vi "Sellafield_Stack_Changeover.vi"(3 "Mode":T5, 5 "Traverse line In":T2 {"Row Duration (mins)" format="%#.1f"; "Row No" min=0; "Trace Gas Concentration (%)" min=0.0 format="%#.2f"; "Emission Rate (l/min)" format="%#.2f"; "Tunnel Speed" format="%#.2f"; "Start X" format="%#.2f"; "Start Y" format="%#.2f"; "Start Z" format="%#.2f"; "End X" format="%#.2f"; "End Y" format="%#.2f"; "End Z" format="%#.2f"; "Averaging time (min)" min=0.0 format="%#.2f"}) -> (0 "Error Message":string, 1 "Status":T1, 2 "Traverse line Out":T2 {"Row Duration (mins)" format="%#.1f"; "Row No" min=0; "Trace Gas Concentration (%)" min=0.0 format="%#.2f"; "Emission Rate (l/min)" format="%#.2f"; "Tunnel Speed" format="%#.2f"; "Start X" format="%#.2f"; "Start Y" format="%#.2f"; "Start Z" format="%#.2f"; "End X" format="%#.2f"; "End Y" format="%#.2f"; "End Z" format="%#.2f"; "Averaging time (min)" min=0.0 format="%#.2f"})   [LabVIEW 2010]
uses:
  Gen Trav/Traverse_cluster.ctl
  Gen Trav/Spacing.ctl
  Controls/Multi_run_mode.ctl
  Controls/User_Specific_mode.ctl
  Gen Trav/Multi_Run_Status.ctl
  ADAM Client/Sub VIs/ADAM Controls/Update_scan_value.ctl
panel:
  # "X           Y            Z"
  # "Start"
  # "End"
  # "X           Y            Z"
  # "Start"
  # "End"
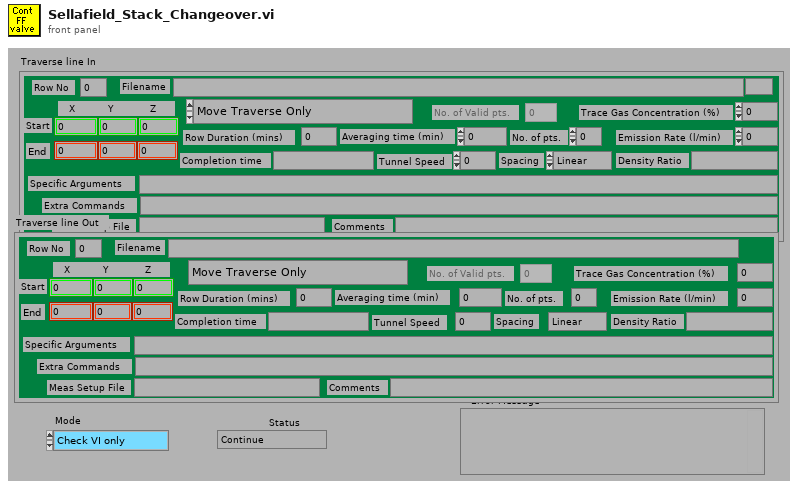
[diagram p1: front panel]
types:
  T1 = typedef "Multi_Run_Status.ctl" = enum16{"Continue", "Jump to Next Point", "Jump to Next Row", "Jump To Fall Back", "Terminate Run"}
  T2 = typedef "Traverse_cluster.ctl" = cluster{"Start X":dbl, "Start Y":dbl, "Start Z":dbl, "End X":dbl, "End Y":dbl, "End Z":dbl, "No. of pts.":i32, "Spacing":T3, "Filename":path, "Tunnel Speed":dbl, "Averaging time (min)":dbl, "Extra Commands":string, "Specific Arguments":string, "Emission Rate (l/min)":dbl, "Trace Gas Concentration (%)":dbl, "Density Ratio":string, "Comments":string, "Row No":i32, "Row Type Selector":T4, "Completion time":string, "Row Duration (mins)":dbl, "No. of Valid pts.":i32, "Meas Setup File":string}
  T3 = typedef "Spacing.ctl" = enum16{"Linear", "Log", "Gauss", "Specified", "N/A"}
  T4 = typedef "Multi_run_mode.ctl" = enum16{"Move Traverse Only", "Set Tunnel Speed Only", "Set Source Only", "Set Measurement Conditions", "Single Measurement", "Vertical Profile", "Lateral Profile", "Longitudinal Profile", "Explore Volume", "Multi-Axis Profile", "Auto Calibrate", "Meas Fast FID Bkgnd", "Check Beam Power", "Scanning Valve Measurement", "Run VI Named:", "Set ADAM Ch", "Wait (minutes)", "Send Message", "Synchronize With:", "Fall Back to this Row", "Turn Off Row Repeating", "Blank Row"}
  T5 = typedef "User_Specific_mode.ctl" = enum16{"Check VI only", "Run VI"}
  T6 = typedef "Update_scan_value.ctl" = cluster{"Channel Name":string, "New Value":dbl}
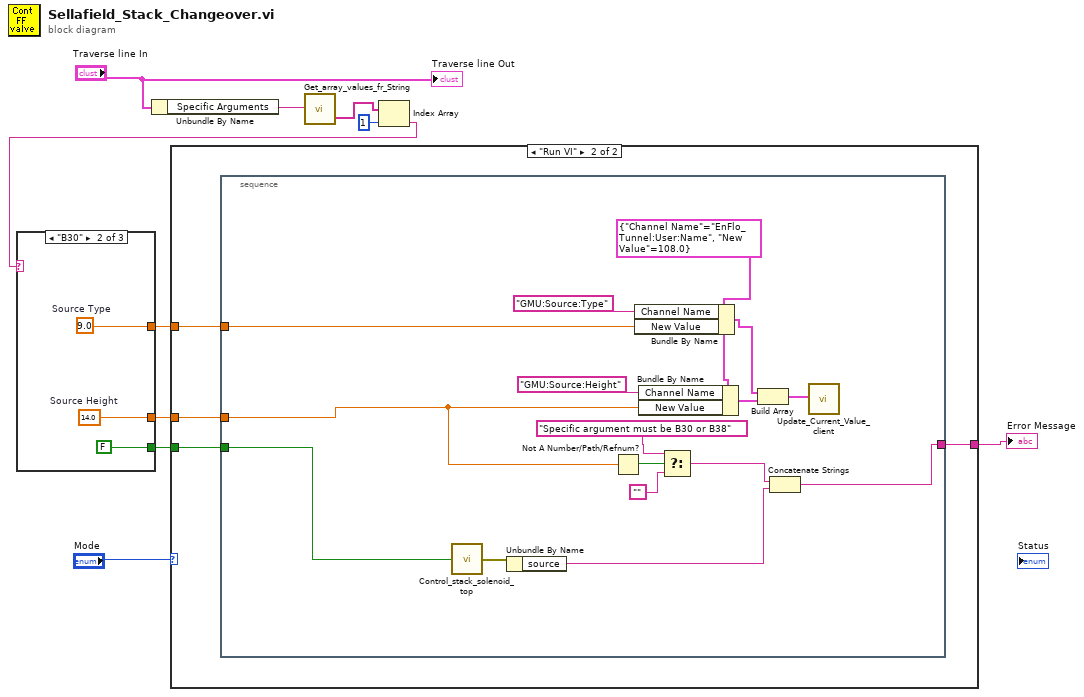
[diagram p0: block diagram]
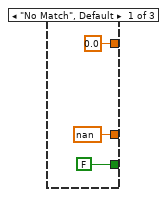
[diagram p2: hidden frame]
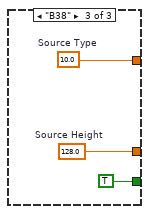
[diagram p3: hidden frame]
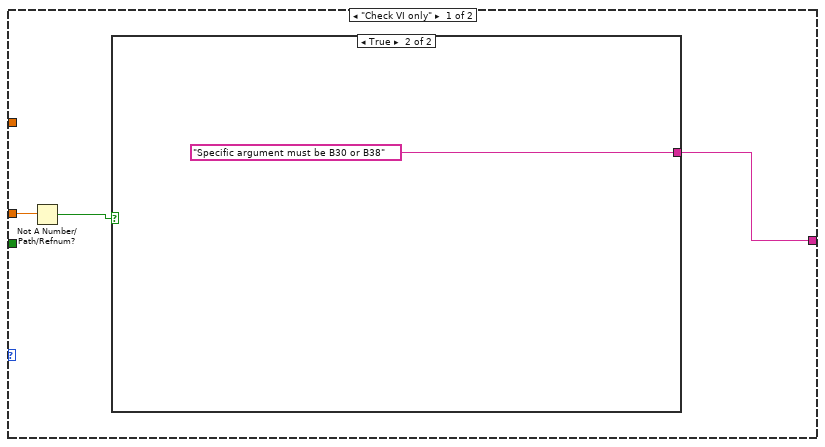
[diagram p4: hidden frame]
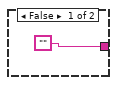
[diagram p5: hidden frame]
diagram:
  n1 = Unbundle By Name("Traverse line In") -> ("Specific Arguments"=w8:string)
  n2 = call "Get_array_values_fr_String.vi"("String Value"=w8) -> ("String array"=w7:string[])  [unwired: 1 out]
  n3 = Index Array(array=w7, index=1 ("Index")) -> (element=w5:string)
  n4 = case shown="\"B30\"" w5 {
    tunnel: [nan ("Source Height") w16 w19] -> w4
    tunnel: [0.0 ("Source Type") w15 w18] -> w3
    tunnel: [FALSE FALSE TRUE] -> w1
    frame "No Match", Default {
    }
    frame "B30" {
      w15 = 9.0  # Source Type
      w16 = 14.0  # Source Height
    }
    frame "B38" {
      w18 = 10.0  # Source Type
      w19 = 128.0  # Source Height
    }
  }
  n5 = case shown="\"Run VI\"" "Mode" {
    tunnel: w4 -> [w22 w28]
    tunnel: w3 -> [_ w27]
    tunnel: [w20 w25] -> w2
    tunnel: w1 -> [_ w26]
    frame "Check VI only" {
      n6 = Not A Number/Path/Refnum?(number/path/refnum=w22) -> (NaN/Path/Refnum?=w21:bool)
      n7 = case shown="True" w21 {
        tunnel: ["" "Specific argument must be B30 or B38"] -> w20
        frame False {
        }
        frame True {
        }
      }
    }
    frame "Run VI" {
      n8 = stacked-sequence {
        tunnel: w28 -> [w35]
        tunnel: w27 -> [w38]
        tunnel: w26 -> [w33]
        tunnel: [w29] -> w25
        frame #0 {
          w39 = T6 {"Channel Name"="EnFlo_Tunnel:User:Name", "New Value"=108.0} ("Update Scan Value Cluster")
          n9 = call "Control_stack_solenoid_top.vi"("Valve On?"=w33) -> ("s? t:f"=w32:errorcluster)  [unwired: 1 out]
          n10 = Unbundle By Name(w32) -> ("source"=w30:string)
          n11 = Not A Number/Path/Refnum?(number/path/refnum=w35) -> (NaN/Path/Refnum?=w36:bool)
          n12 = Bundle By Name(cluster=w39, "Channel Name"="GMU:Source:Type", "New Value"=w38) -> (w40:T6)
          n13 = Bundle By Name(cluster=w39, "Channel Name"="GMU:Source:Height", "New Value"=w35) -> (w42:T6)
          n14 = Select(t="Specific argument must be B30 or B38", s=w36, f="") -> (s? t:f=w31:string)
          n15 = Build Array(w40, w42) -> (w43:T6[])
          n16 = Concatenate Strings(w31, w30) -> (w29:string)
          n17 = call "Update_Current_Value_client.vi"("Update array in"=w43) -> ()  [unwired: 1 in]
        }
      }
    }
  }
  "Error Message" <- w2
  "Traverse line Out" <- "Traverse line In"
